vi "VI Anlagengrenzwerte Amium.vi"() -> ()   [LabVIEW 2015, in "PNS.lvlib"]
uses:
  PNS/PNS.lvlib
  PNS/Anlagengrenzwerte PNS.ctl
  PNS/Anlagengrenzwerte-Parameter Anzeige.ctl
  Visualisierungs Elemente/Zahlen-Eingabefeld.ctl
  Visualisierungs Elemente/Button.ctl
  Visualisierungs Elemente/Zahlen-Ausgabefeld.ctl
  PNS/PNS Istwerte.ctl
  PNS/Aktionen FGV Grenzwerte.ctl
  PNS/Aktionen FGV Loopkennung.ctl
  PNS/PNS Anlagenuebersicht einfaerben Aktionen.ctl
  Amium PNS/Aktion FGV Amium Daten.ctl
  Passwortverwaltung/FGV Passwort Aktion.ctl
  PNS/Komm Modbus/Aktionen FGV Komm MB.ctl
  PNS/Aktionen FGV Istwerte.ctl
  PNS/Diagnose PNS.vi
  Passwortverwaltung/Passwort.lvlib
  Allgemein/allgemeine Sub-VIs.lvlib
  PNS/Komm Modbus/Modbus TypDef.lvlib
  PNS/Komm Modbus/Komm Modbus.lvlib
  Amium PNS/Amium PNS.lvlib
panel:
  in  "IP-Adresse PNS:":string
  in  "Port":u16
  out "Software Version:":string
  out "PNS Istwerte":T1 {"Istwert 8" format="%.1f"; "Istwert 7" format="%.1f"; "Istwert 6" format="%.1f"; "Istwert 5" format="%.1f"; "Istwert 4" format="%.1f"; "Istwert 3" format="%.1f"; "Istwert 2" format="%.1f"; "Istwert 1" format="%.1f"}
  out "Seriennummer:":string
  out "Gerätetyp:":string
  out "Detail Status:":T2 format="%#_5g"
  out "Status:":T2 format="%#_5g"
  out "Druckluft Störung:":T2 format="%#_5g"
  out "AWC IST:":T2 format="%#_5g"
  out "AWC Soll:":T2 format="%#_5g"
  out "Error Out":errorcluster caption="Fehlercluster"
  in  "Diag PNS":T3
  in  "Grenzwerte PNS":T4={"Filter:"={"Sollwert"=0.0, "Warn-Min"=0.0, "Warn-Max"=0.0, "Abschalt-Min"=0.0, "Abschalt-Max"=0.0, "Regler"=1, "AnlagenParameter"=""}, "Ventilplatte:"={"Sollwert"=0.0, "Warn-Min"=0.0, "Warn-Max"=0.0, "Abschalt-Min"=0.0, "Abschalt-Max"=0.0, "Regler"=1, "AnlagenParameter"=""}, "Heizleitung 1:"={"Sollwert"=0.0, "Warn-Min"=0.0, "Warn-Max"=0.0, "Abschalt-Min"=0.0, "Abschalt-Max"=0.0, "Regler"=1, "AnlagenParameter"=""}, "Heizleitung 2:"={"Sollwert"=0.0, "Warn-Min"=0.0, "Warn-Max"=0.0, "Abschalt-Min"=0.0, "Abschalt-Max"=0.0, "Regler"=1, "AnlagenParameter"=""}, "Heizleitung 3:"={"Sollwert"=0.0, "Warn-Min"=0.0, "Warn-Max"=0.0, "Abschalt-Min"=0.0, "Abschalt-Max"=0.0, "Regler"=1, "AnlagenParameter"=""}, "Heizleitung 4:"={"Sollwert"=0.0, "Warn-Min"=0.0, "Warn-Max"=0.0, "Abschalt-Min"=0.0, "Abschalt-Max"=0.0, "Regler"=1, "AnlagenParameter"=""}, "Heizleitung 5:"={"Sollwert"=0.0, "Warn-Min"=0.0, "Warn-Max"=0.0, "Abschalt-Min"=0.0, "Abschalt-Max"=0.0, "Regler"=1, "AnlagenParameter"=""}, "Heizleitung 6:"={"Sollwert"=0.0, "Warn-Min"=0.0, "Warn-Max"=0.0, "Abschalt-Min"=0.0, "Abschalt-Max"=0.0, "Regler"=1, "AnlagenParameter"=""}} {"Heizleitung 6:"."Regler" items=["aktiv", "inaktiv"]; "Heizleitung 6:"."Abschalt-Max" format="%#_5g"; "Heizleitung 6:"."Abschalt-Min" format="%#_5g"; "Heizleitung 6:"."Warn-Max" format="%#_5g"; "Heizleitung 6:"."Warn-Min" format="%#_5g"; "Heizleitung 6:"."Sollwert" format="%#_5g"; "Heizleitung 5:"."Regler" items=["aktiv", "inaktiv"]; "Heizleitung 5:"."Abschalt-Max" format="%#_5g"; "Heizleitung 5:"."Abschalt-Min" format="%#_5g"; "Heizleitung 5:"."Warn-Max" format="%#_5g"; "Heizleitung 5:"."Warn-Min" format="%#_5g"; "Heizleitung 5:"."Sollwert" format="%#_5g"; "Heizleitung 4:"."Regler" items=["aktiv", "inaktiv"]; "Heizleitung 4:"."Abschalt-Max" format="%#_5g"; "Heizleitung 4:"."Abschalt-Min" format="%#_5g"; "Heizleitung 4:"."Warn-Max" format="%#_5g"; "Heizleitung 4:"."Warn-Min" format="%#_5g"; "Heizleitung 4:"."Sollwert" format="%#_5g"; "Heizleitung 3:"."Regler" items=["aktiv", "inaktiv"]; "Heizleitung 3:"."Abschalt-Max" format="%#_5g"; "Heizleitung 3:"."Abschalt-Min" format="%#_5g"; "Heizleitung 3:"."Warn-Max" format="%#_5g"; "Heizleitung 3:"."Warn-Min" format="%#_5g"; "Heizleitung 3:"."Sollwert" format="%#_5g"; "Heizleitung 2:"."Regler" items=["aktiv", "inaktiv"]; "Heizleitung 2:"."Abschalt-Max" format="%#_5g"; "Heizleitung 2:"."Abschalt-Min" format="%#_5g"; "Heizleitung 2:"."Warn-Max" format="%#_5g"; "Heizleitung 2:"."Warn-Min" format="%#_5g"; "Heizleitung 2:"."Sollwert" format="%#_5g"; "Heizleitung 1:"."Regler" items=["aktiv", "inaktiv"]; "Heizleitung 1:"."Abschalt-Max" format="%#_5g"; "Heizleitung 1:"."Abschalt-Min" format="%#_5g"; "Heizleitung 1:"."Warn-Max" format="%#_5g"; "Heizleitung 1:"."Warn-Min" format="%#_5g"; "Heizleitung 1:"."Sollwert" format="%#_5g"; "Ventilplatte:"."Regler" items=["aktiv", "inaktiv"]; "Ventilplatte:"."Abschalt-Max" format="%#_5g"; "Ventilplatte:"."Abschalt-Min" format="%#_5g"; "Ventilplatte:"."Warn-Max" format="%#_5g"; "Ventilplatte:"."Warn-Min" format="%#_5g"; "Ventilplatte:"."Sollwert" format="%#_5g"; "Filter:"."Regler" items=["aktiv", "inaktiv"]; "Filter:"."Abschalt-Max" format="%#_5g"; "Filter:"."Abschalt-Min" format="%#_5g"; "Filter:"."Warn-Max" format="%#_5g"; "Filter:"."Warn-Min" format="%#_5g"; "Filter:"."Sollwert" format="%#_5g"}
  # "Anlagengrenzwerte PNS"
  # "Abschaltgrenzen"
  # "Warngrenzen"
  # "Regelung \naktiv/inaktiv"
  # "Parameter"
  # "Istwert"
  # "Sollwert"
  # "Min"
  # "Max"
  # "Min"
  # "Max"
  # "Allgemeine Werte"
  # "Status Kommunikation"
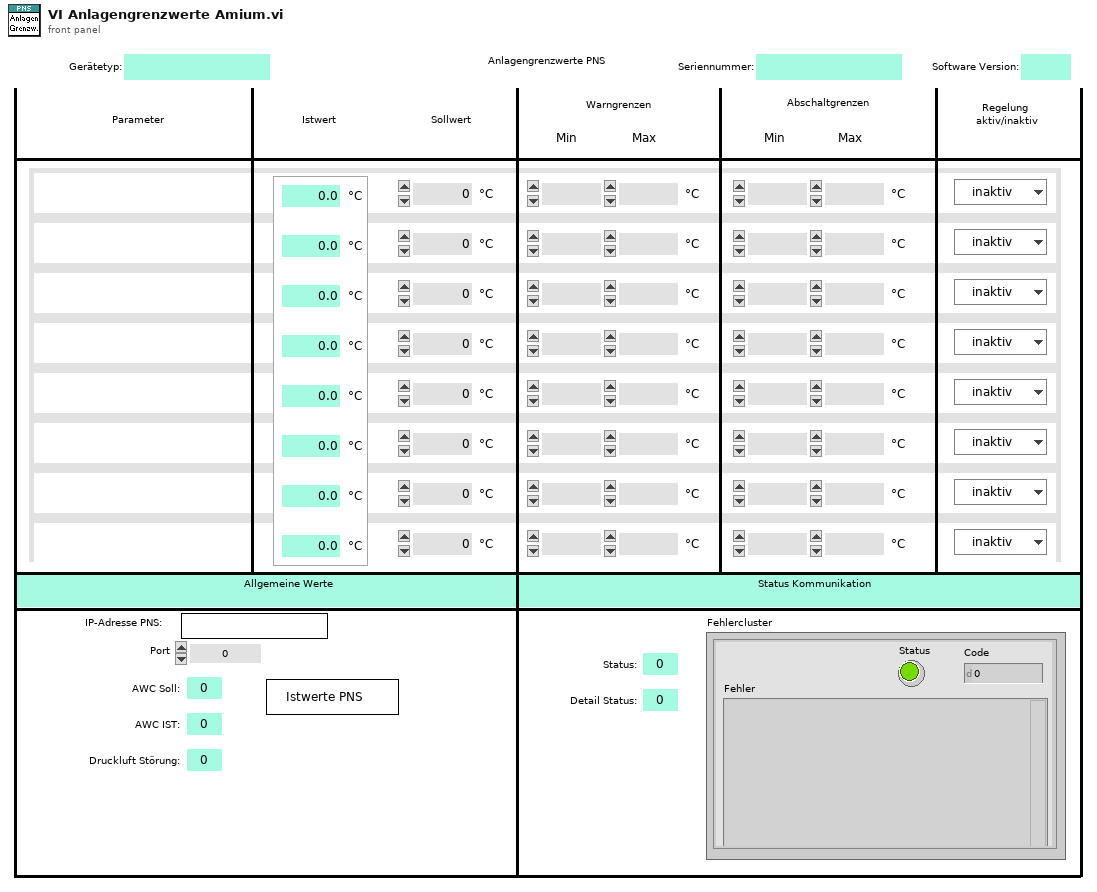
[diagram p1: front panel]
types:
  T1 = typedef "PNS.lvlib/PNS Istwerte.ctl" = cluster{"Istwert 1":sgl, "Istwert 2":sgl, "Istwert 3":sgl, "Istwert 4":sgl, "Istwert 5":sgl, "Istwert 6":sgl, "Istwert 7":sgl, "Istwert 8":sgl}
  T2 = typedef "Zahlen-Ausgabefeld.ctl" = sgl
  T3 = typedef "Button.ctl" = bool
  T4 = typedef "PNS.lvlib/Anlagengrenzwerte PNS.ctl" = cluster{"Filter:":T5, "Ventilplatte:":T5, "Heizleitung 1:":T5, "Heizleitung 2:":T5, "Heizleitung 3:":T5, "Heizleitung 4:":T5, "Heizleitung 5:":T5, "Heizleitung 6:":T5}
  T5 = typedef "PNS.lvlib/Anlagengrenzwerte-Parameter Anzeige.ctl" = cluster{"Sollwert":T6, "Warn-Min":T6, "Warn-Max":T6, "Abschalt-Min":T6, "Abschalt-Max":T6, "Regler":u16, "AnlagenParameter":string}
  T6 = typedef "Zahlen-Eingabefeld.ctl" = sgl
  T7 = typedef "Amium PNS.lvlib/Aktion FGV Amium Daten.ctl" = enum16{"lesen", "Komm Daten", "Daten", "Error", "Regler", "Grenzwerte", "laden", "speichern"}
  T8 = typedef "PNS.lvlib/PNS Anlagenuebersicht einfaerben Aktionen.ctl" = enum16{"lesen", "prüfen", "initialisieren"}
  T9 = typedef "PNS.lvlib/Aktionen FGV Loopkennung.ctl" = enum16{"lesen", "schreiben"}
  T10 = typedef "PNS.lvlib/Aktionen FGV Grenzwerte.ctl" = enum16{"lesen", "Grenzw. schreiben", "Anweisungscode", "IP-Adresse"}
  T11 = cluster{"Loops":string[], "Gerätetype":string, "Loopkennung":u16[], "Seriennummer":string, "Geraetekennung":u16, "SoftWare Version":string}
  T12 = typedef "Amium PNS.lvlib/Kommunikation Daten Cluster.ctl" = cluster{"IP Adresse":string, "Port":i16}
  T13 = typedef "Passwort.lvlib/FGV Passwort Aktion.ctl" = enum16{"prüfen", "setzen", "Initialisieren", "PW speichern", "lesen", "PW Änderung"}
  T14 = typedef "PNS.lvlib/Aktionen FGV Istwerte.ctl" = enum16{"lesen", "initialisieren", "schreiben", "Störungen"}
  T15 = typedef "PNS.lvlib/Komm Modbus.lvlib/Modbus TypDef.lvlib/Aktionen FGV Komm MB.ctl" = enum16{"initialisieren", "lesen", "Verbindung herstellen", "Verbindung beenden", "Komm Modbus", "Sollwerte vorgeben", "change lang"}
  T16 = typedef "Steuerung PNS.lvclass/Regler.ctl" = cluster{"Istwert":i16, "Sollwert":i16, "Alarm MIN":i16, "Alarm MAX":i16, "Regler sperren":i16, "Analog Ausgang":i16}[]
  T17 = cluster{"Istwert":i16, "Sollwert":i16, "Alarm MIN":i16, "Alarm MAX":i16, "Regler sperren":i16, "Analog Ausgang":i16}
  T18 = cluster{"Istwert":i16, "Istwert":i16, "Istwert":i16, "Istwert":i16, "Istwert":i16, "Istwert":i16, "Istwert":i16, "Istwert":i16}
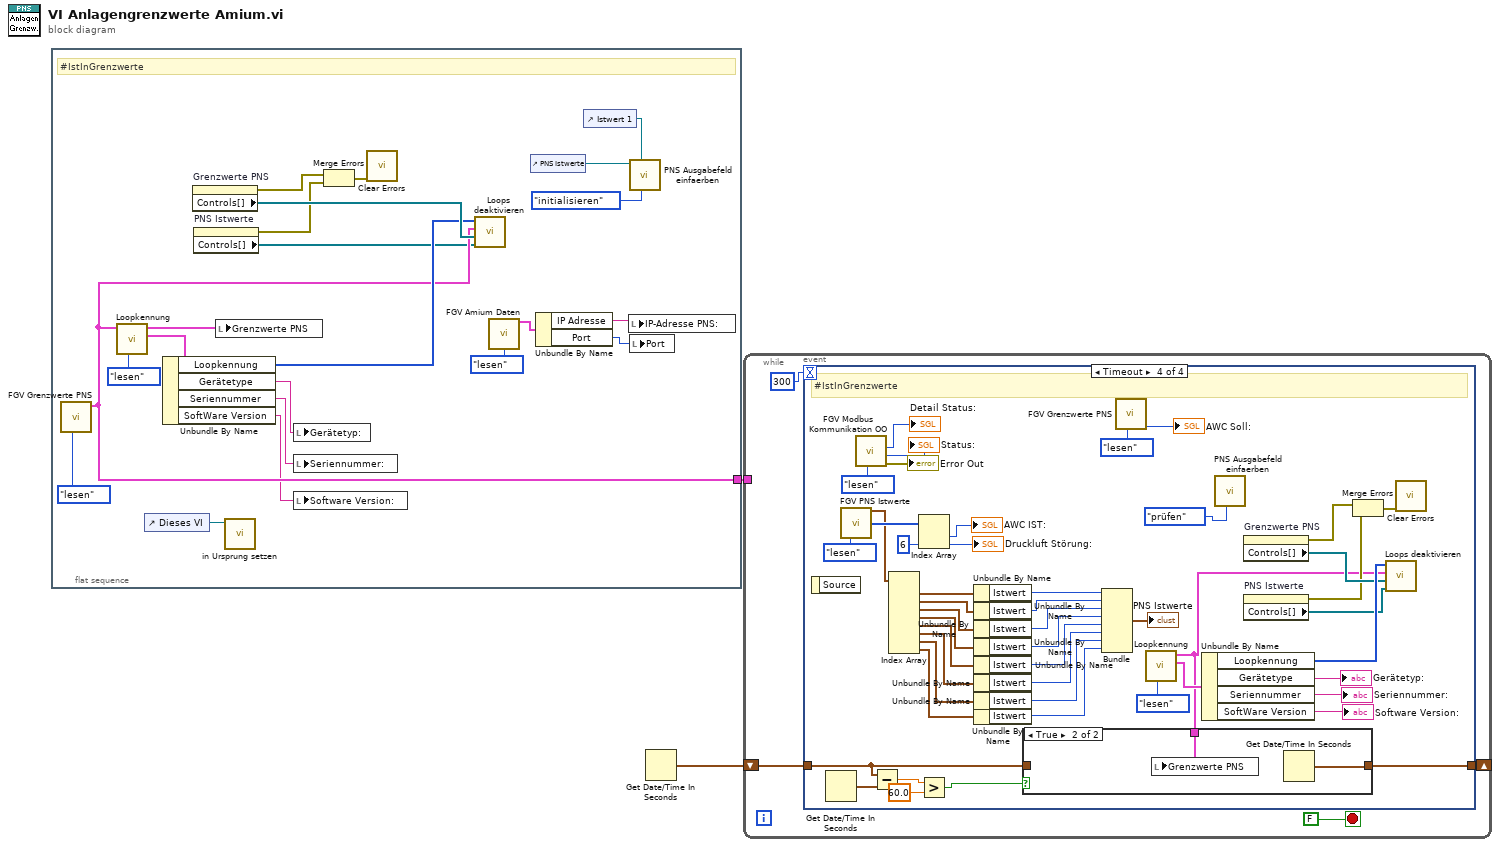
[diagram p0: block diagram]
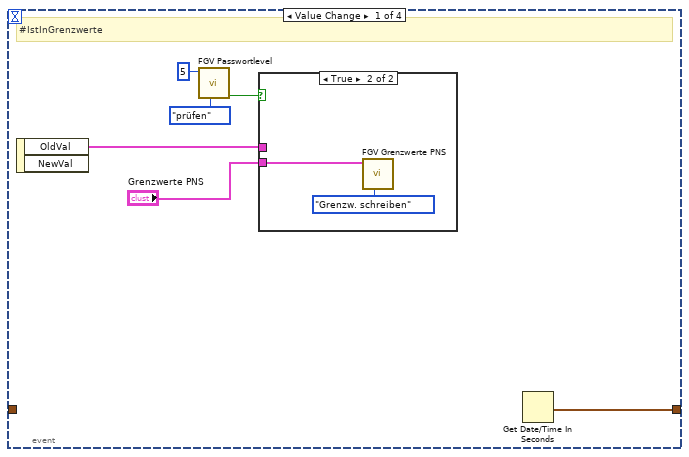
[diagram p2: hidden frame]
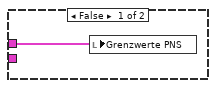
[diagram p3: hidden frame]
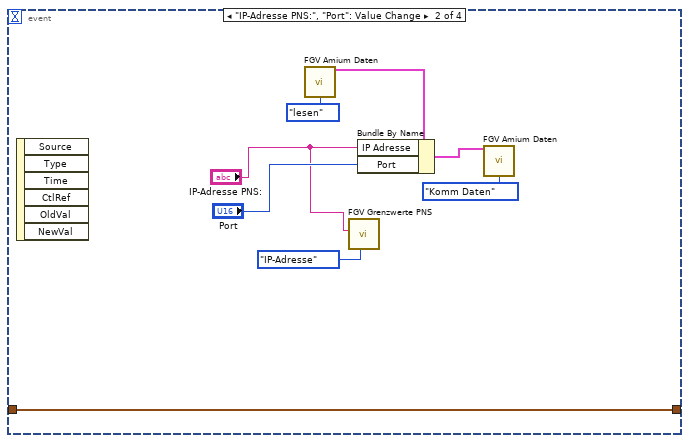
[diagram p4: hidden frame]
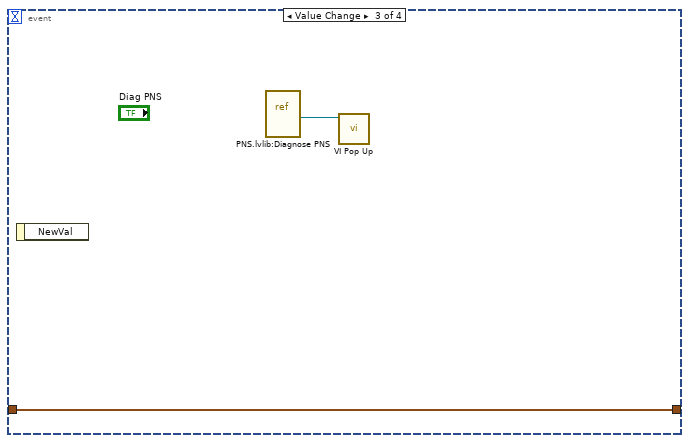
[diagram p5: hidden frame]
diagram:
  n1 = flat-sequence {
    tunnel: [w15] -> w2
    frame #0 {
      # "#IstInGrenzwerte"
      n2 = call "FGV Grenzwerte PNS.vi"("Aktionen FGV Grenzwerte"=Aktionen_FGV_Grenzwerte."lesen") -> ("Grenzwerte PNS"=w15:T4)  [unwired: 8 in, 2 out]
      n3 = call "Loopkennung.vi"("Aktion"=Aktionen_FGV_Loopkennung."lesen", "Grenzwerte PNS"=w15) -> ("LoopGeraetekennung"=w20:T11, "Grenzwerte PNS"=w22:T4)  [unwired: 8 in]
      n4 = control-ref of="Dieses VI"() -> (w23:refnum<vi>)
      n5 = Unbundle By Name(w20) -> ("Loopkennung"=w16:u16[], "Gerätetype"=w19:string, "Seriennummer"=w18:string, "SoftWare Version"=w13:string)
      n6 = property on="Grenzwerte PNS" class="Cluster (strikt)"() -> (error out=w10:errorcluster, "Controls[]"=w17:refnum<vi>[])  [unwired: 2 in, 1 out]
      n7 = property on="PNS Istwerte" class="Cluster (strikt)"() -> (error out=w11:errorcluster, "Controls[]"=w12:refnum<vi>[])  [unwired: 2 in, 1 out]
      n8 = local write "Grenzwerte PNS"(w22) -> ()
      n9 = call "in Ursprung setzen.vi"("VI Referenz"=w23) -> ()  [unwired: 11 in]
      n10 = local write "Gerätetyp:"(w19) -> ()
      n11 = local write "Seriennummer:"(w18) -> ()
      n12 = local write "Software Version:"(w13) -> ()
      n13 = Merge Errors(w10, w11) -> (w14:errorcluster)
      n14 = call <vilib>:"Clear Errors.vi"("error in (no error)"=w14) -> ()  [unwired: 5 in, 2 out]
      n15 = call "Loops deaktivieren.vi"("Istwert Controls[]"=w12, "Grenzwert Controls[]"=w17, "Grenzwerte PNS"=w15, "Loopkennung"=w16) -> ()  [unwired: 8 in]
      n16 = call "FGV Amium Daten.vi"("Aktion"=Aktion_FGV_Amium_Daten."lesen") -> ("Amium Komm Daten"=w5:T12)  [unwired: 9 in, 5 out]
      n17 = control-ref of="PNS Istwerte"() -> (w8:refnum<vi>)
      n18 = Unbundle By Name(w5) -> ("IP Adresse"=w4:string, "Port"=w3:i16)
      n19 = control-ref of="Istwert 1"() -> (w7:refnum<vi>)
      n20 = local write "IP-Adresse PNS:"(w4) -> ()
      n21 = call "PNS Ausgabefeld einfaerben.vi"("Aktionen"=PNS_Anlagenuebersicht_einfaerben_Aktionen."initialisieren", "FeldTyp (Eingang)"=w7, "PNS Istwerte"=w8) -> ()  [unwired: 9 in]
      n22 = local write "Port"(w3) -> ()
    }
  }
  n23 = Get Date/Time In Seconds() -> (seconds since 1Jan1904=w1:timestamp)
  n24 = while {
    tunnel: w2 -> [_]
    shift-right: [w25] -> _
    shift-left: w1 -> [w26]
    stop <- FALSE stop-if-true
    n25 = event shown="[3] Timeout" {
      selector: _ -> [_ _ _ _]
      dyn-events: _ -> [_ _ _ _]
      timeout: 300 -> [_ _ _ _]
      tunnel: w26 -> [_ w44 w46 w62]
      tunnel: [w29 w44 w46 w61] -> w25
      event Value Change {
        # "#IstInGrenzwerte"
        n26 = event-data() -> ("OldVal"=w31:T4)  [unwired: 2 out]
        n27 = call "FGV Passwortlevel.vi"("FGV Passwort Aktion"=FGV_Passwort_Aktion."prüfen", "geforderter Level"=i16 5) -> ("Freigabe"=w32:bool)  [unwired: 2 in, 7 out]
        n28 = case shown="True" w32 {
          tunnel: "Grenzwerte PNS" -> [_ w36]
          tunnel: w31 -> [w35 _]
          frame False {
            n29 = local write "Grenzwerte PNS"(w35) -> ()
          }
          frame True {
            n30 = call "FGV Grenzwerte PNS.vi"("Aktionen FGV Grenzwerte"=Aktionen_FGV_Grenzwerte."Grenzw. schreiben", "Grenzwerte PNS"=w36) -> ()  [unwired: 7 in, 3 out]
          }
        }
        n31 = Get Date/Time In Seconds() -> (seconds since 1Jan1904=w29:timestamp)
      }
      event "IP-Adresse PNS:", "Port": Value Change {
        n32 = event-data() -> ()  [unwired: 7 out]
        n33 = call "FGV Amium Daten.vi"("Aktion"=Aktion_FGV_Amium_Daten."lesen") -> ("Amium Komm Daten"=w42:T12)  [unwired: 9 in, 5 out]
        n34 = call "FGV Grenzwerte PNS.vi"("Aktionen FGV Grenzwerte"=Aktionen_FGV_Grenzwerte."IP-Adresse", "IP-Adresse"="IP-Adresse PNS:") -> ()  [unwired: 7 in, 3 out]
        n35 = Bundle By Name(cluster=w42, "IP Adresse"="IP-Adresse PNS:", "Port"="Port") -> (w40:T12)
        n36 = call "FGV Amium Daten.vi"("Amium Komm  Daten"=w40, "Aktion"=Aktion_FGV_Amium_Daten."Komm Daten") -> ()  [unwired: 8 in, 6 out]
      }
      event Value Change {
        n37 = event-data() -> ()  [unwired: 2 out]
        n38 = vi-ref "PNS.lvlib:Diagnose PNS.vi"() -> (w47:refnum<vi>)
        n39 = call "VI Pop Up.vi"("VI Referenz"=w47) -> ()  [unwired: 11 in]
      }
      event Timeout {
        # "#IstInGrenzwerte"
        n40 = event-data() -> ()  [unwired: 2 out]
        n41 = Get Date/Time In Seconds() -> (seconds since 1Jan1904=w66:timestamp)
        n42 = call "FGV PNS Istwerte.vi"("Aktionen"=Aktionen_FGV_Istwerte."lesen") -> ("Regler"=w67:T16, "UsrVal"=w85:u16[])  [unwired: 11 in, 2 out]
        n43 = call "FGV Modbus Kommunikation OO.vi"("Aktionen"=Aktionen_FGV_Komm_MB."lesen") -> ("Fehler (Ausgang)"=→"Error Out":errorcluster, "Index"=→"Status:":u8, "Case Nr."=→"Detail Status:":u8)  [unwired: 5 in, 1 out]
        n44 = Subtract(x=w62, y=w66) -> (x-y=w65:dbl)
        n45 = Index Array(array=w67) -> (element #1=w84:T17, element #2=w83:T17, element #3=w82:T17, element #4=w80:T17, element #5=w81:T17, element #6=w79:T17, element #7=w78:T17, element #8=w70:T17)  [unwired: 8 in]
        n46 = Index Array(array=w85, index #2=6 ("Index")) -> (element #1=→"AWC IST:":u16, element #2=→"Druckluft Störung:":u16)  [unwired: 1 in]
        n47 = Greater?(x=w65, y=60.0) -> (0:w63:bool)
        n48 = Unbundle By Name(w84) -> ("Istwert"=w77:i16)
        n49 = Unbundle By Name(w83) -> ("Istwert"=w76:i16)
        n50 = Unbundle By Name(w82) -> ("Istwert"=w75:i16)
        n51 = Unbundle By Name(w80) -> ("Istwert"=w74:i16)
        n52 = Unbundle By Name(w81) -> ("Istwert"=w73:i16)
        n53 = Unbundle By Name(w79) -> ("Istwert"=w72:i16)
        n54 = Unbundle By Name(w78) -> ("Istwert"=w71:i16)
        n55 = Unbundle By Name(w70) -> ("Istwert"=w69:i16)
        n56 = Bundle("Istwert"=w77, "Istwert"=w76, "Istwert"=w75, "Istwert"=w74, "Istwert"=w73, "Istwert"=w72, "Istwert"=w71, "Istwert"=w69) -> (→"PNS Istwerte":T18)  [unwired: 1 in]
        n57 = call "FGV Grenzwerte PNS.vi"("Aktionen FGV Grenzwerte"=Aktionen_FGV_Grenzwerte."lesen") -> ("Anweisungscode"=→"AWC Soll:":u16)  [unwired: 8 in, 2 out]
        n58 = call "Loopkennung.vi"("Aktion"=Aktionen_FGV_Loopkennung."lesen") -> ("LoopGeraetekennung"=w59:T11, "Grenzwerte PNS"=w49:T4)  [unwired: 9 in]
        n59 = case shown="True" w63 {
          tunnel: w62 -> [w96 _]
          tunnel: [w96 w98] -> w61
          tunnel: w49 -> [_ w97]
          frame False {
          }
          frame True {
            n60 = local write "Grenzwerte PNS"(w97) -> ()
            n61 = Get Date/Time In Seconds() -> (seconds since 1Jan1904=w98:timestamp)
          }
        }
        n62 = Unbundle By Name(w59) -> ("Loopkennung"=w55:u16[], "Gerätetype"=→"Gerätetyp:":string, "Seriennummer"=→"Seriennummer:":string, "SoftWare Version"=→"Software Version:":string)
        n63 = call "PNS Ausgabefeld einfaerben.vi"("Aktionen"=PNS_Anlagenuebersicht_einfaerben_Aktionen."prüfen") -> ()  [unwired: 11 in]
        n64 = property on="Grenzwerte PNS" class="Cluster (strikt)"() -> (error out=w51:errorcluster, "Controls[]"=w53:refnum<vi>[])  [unwired: 2 in, 1 out]
        n65 = property on="PNS Istwerte" class="Cluster (strikt)"() -> (error out=w50:errorcluster, "Controls[]"=w54:refnum<vi>[])  [unwired: 2 in, 1 out]
        n66 = Merge Errors(w51, w50) -> (w52:errorcluster)
        n67 = call "Loops deaktivieren.vi"("Istwert Controls[]"=w54, "Grenzwert Controls[]"=w53, "Grenzwerte PNS"=w49, "Loopkennung"=w55) -> ()  [unwired: 8 in]
        n68 = call <vilib>:"Clear Errors.vi"("error in (no error)"=w52) -> ()  [unwired: 5 in, 2 out]
      }
    }
  }
